vi "Symphony Wavelght Conver.vi"(4 "Angle Y (deg)":dbl=12.5 format="%#_13g", 6 "Focale":dbl=320.0 format="%#_13g", 7 "PixelArr":ext[](array[numeric]), 8 "error in (no error)":errorcluster, 9 "Angle D(deg)":dbl=21.26 format="%#_13g", 10 "Lambda":dbl, 11 "Grooves(l/mm)":dbl=1800.0 format="%#_13g") -> (0 "error out":errorcluster, 3 "Tableau":dbl[](array[numeric]))   [LabVIEW 2019]
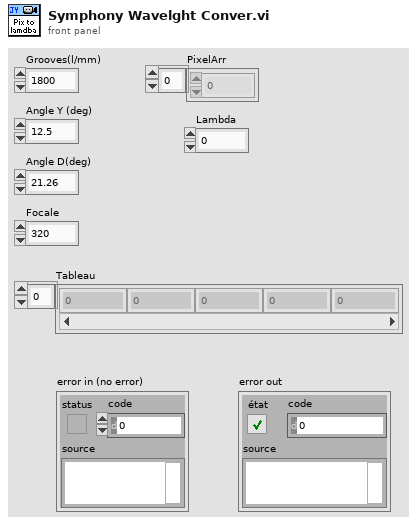
[diagram p1: front panel]
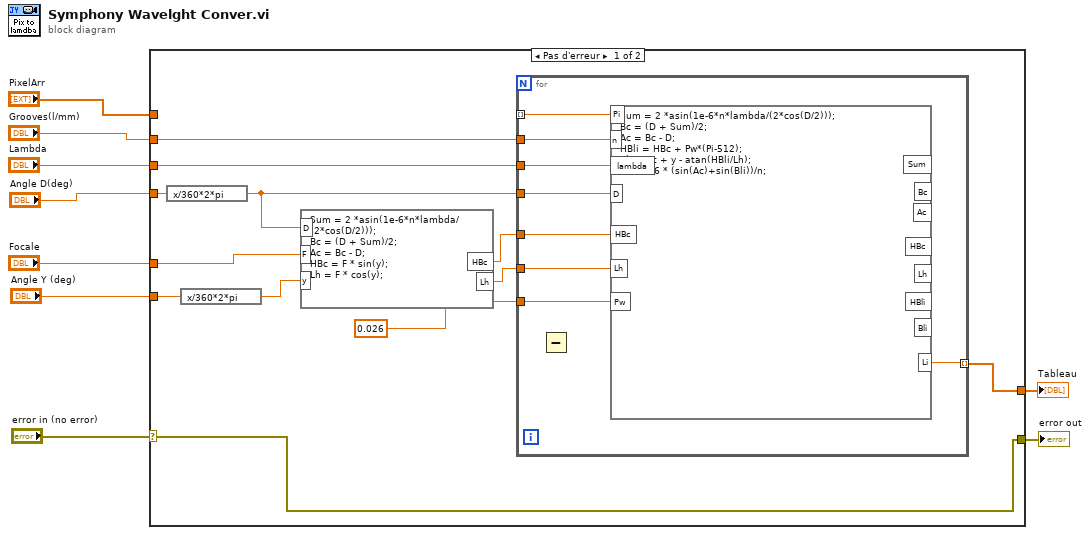
[diagram p0: block diagram]
diagram:
  n1 = case shown="Pas d'erreur" "error in (no error)" {
    selector: "error in (no error)" -> [w17 w32]
    tunnel: "Grooves(l/mm)" -> [w23 _]
    tunnel: "Focale" -> [w13 _]
    tunnel: "Angle Y (deg)" -> [w16 _]
    tunnel: "Angle D(deg)" -> [w11 _]
    tunnel: "Lambda" -> [w20 _]
    tunnel: "PixelArr" -> [w19 _]
    tunnel: [w18 _] -> w3
    tunnel: [w17 w32] -> w1
    frame No Error {
      n2 = expression code="x/360*2*pi"(w11) -> (w10:dbl)
      n3 = expression code="x/360*2*pi"(w16) -> (w14:dbl)
      n4 = formula code="Sum = 2 *asin(1e-6*n*lambda/(2*cos(D/2)));\nBc = (D + Sum)/2;\nAc = Bc - D;\nHBc = F * sin(y);\nLh = F * cos(y);"("F"=w13, "y"=w14, "D"=w10) -> ("HBc"=w15:dbl, "Lh"=w12:dbl)
      n5 = for {
        tunnel: w23 -> [w31]
        tunnel: w20 -> [w30]
        tunnel: w10 -> [w29]
        tunnel: w15 -> [w28]
        tunnel: w12 -> [w27]
        tunnel: [w25] -> w21 mode=indexing
        tunnel: 0.026 ("variable en entrée") -> [w26]
        tunnel: [w24] -> w18 mode=indexing
        n6 = Subtract() -> ()  [unwired: 2 in, 1 out]
        n7 = formula code="Sum = 2 *asin(1e-6*n*lambda/(2*cos(D/2)));\nBc = (D + Sum)/2;\nAc = Bc - D;\nHBli = HBc + Pw*(Pi-512);\nBli = Bc + y - atan(HBli/Lh);\nLi = 1e6 * (sin(Ac)+sin(Bli))/n;"("n"=w31, "lambda"=w30, "D"=w29, "HBc"=w28, "Lh"=w27, "Pw"=w26, "Pi"=w25) -> ("Li"=w24:dbl)  [unwired: 7 out]
      }
    }
    frame Error {
    }
  }
  "Tableau" <- w3
  "error out" <- w1
